vi "Read Msg.Noti.Ref.vi"(8 "error in (no error)":errorcluster, 11 "Messaging in":refnum<class "Messaging.lvclass">) -> (0 "error out":errorcluster, 2 "Msg.Noti.Ref":T1, 3 "Messaging out":refnum<class "Messaging.lvclass">)   [LabVIEW 2023, in "Messaging.lvclass"]
uses:
  Messaging.lvclass
  Messaging.lvclass/Messaging.ctl
  Msg/Msg.Data.ctl
  Msg/Msg.Noti.Ref.ctl
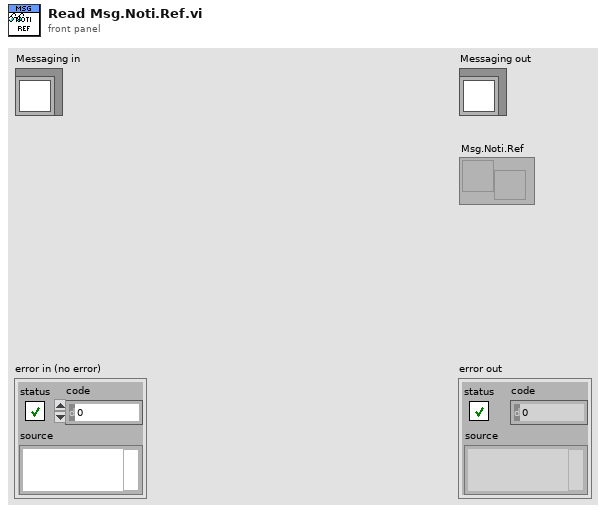
[diagram p1: front panel]
types:
  T1 = typedef "Msg.Noti.Ref.ctl" = refnum<notifier>
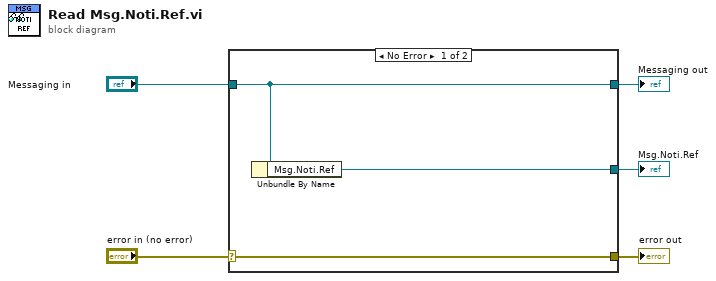
[diagram p0: block diagram]
diagram:
  n1 = case shown="No Error" "error in (no error)" {
    selector: "error in (no error)" -> [w8 w9]
    tunnel: [w8 w9] -> w4
    tunnel: [w7 w10] -> w2
    tunnel: "Messaging in" -> [w7 w10]
    tunnel: [w6 _] -> w1
    frame No Error {
      n2 = Unbundle By Name(w7) -> ("Msg.Noti.Ref"=w6:T1)
    }
    frame Error {
    }
  }
  "error out" <- w4
  "Messaging out" <- w2
  "Msg.Noti.Ref" <- w1
